vi "CurrentAutoModeParameters.vi"(8 "New Auto Mode Parameters":T1={"movementDirection"=enum."TOWARDS_180_DEGREES", "frequency"=1.0}, 11 "Operation":T2) -> (3 "Current Auto Mode Parameters":T1={"movementDirection"=enum."TOWARDS_180_DEGREES", "frequency"=1.0})   [LabVIEW 2024]
uses:
  DataTypes/OperationTypeForFunctionalGlobalVariable.ctl
  DataTypes/AutoModeParameters.ctl
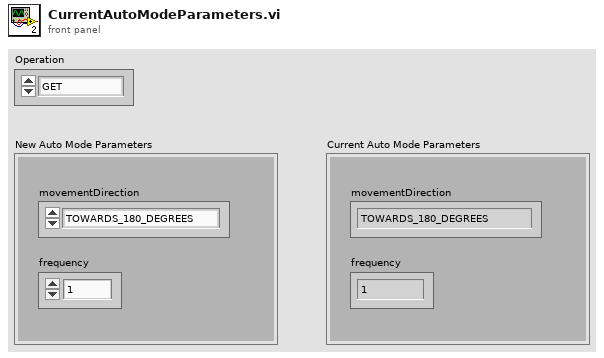
[diagram p1: front panel]
types:
  T1 = typedef "AutoModeParameters.ctl" = cluster{"movementDirection":enum16{"TOWARDS_0_DEGREES", "TOWARDS_180_DEGREES"}, "frequency":dbl}
  T2 = typedef "OperationTypeForFunctionalGlobalVariable.ctl" = enum16{"GET", "SET"}
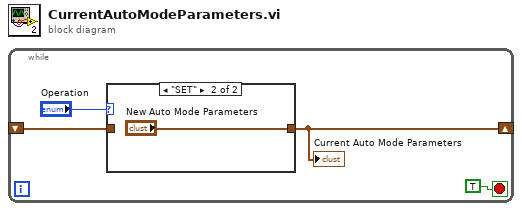
[diagram p0: block diagram]
diagram:
  n1 = while {
    shift-right: [w1] -> _
    shift-left: _ -> [w3]
    stop <- TRUE stop-if-true
    n2 = case shown="\"SET\"" "Operation" {
      tunnel: w3 -> [w5 _]
      tunnel: [w5 "New Auto Mode Parameters"] -> w1
      frame "GET", Default {
      }
      frame "SET" {
      }
    }
    "Current Auto Mode Parameters" <- w1
  }
